vi "IMAQ FPGA Camera Link Data to Pixels 1 Tap 8-Bit.vi"(1 "Camera Link Data":cluster{"Port A":u8}) -> (0 "Pixel":u8)   [LabVIEW 2020]
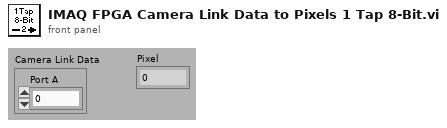
[diagram p1: front panel]
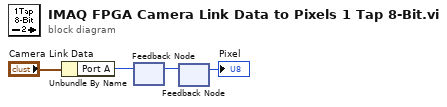
[diagram p0: block diagram]
diagram:
  n1 = Unbundle By Name("Camera Link Data") -> ("Port A"=w3:u8)
  n2 = feedback-in #1(w3) -> ()
  n3 = feedback #1() -> (w2:u8)  [unwired: 1 in]
  n4 = feedback #2() -> (→"Pixel":u8)  [unwired: 1 in]
  n5 = feedback-in #2(w2) -> ()
